vi "_NiFpga_HdlFifo_GetStream.vi"(7 "NUM_DMA_CHANNELS":u32=64, 11 "Fifo Number":u32) -> (3 "Fifo Stream":u32)   [LabVIEW 2023]
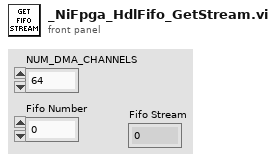
[diagram p1: front panel]
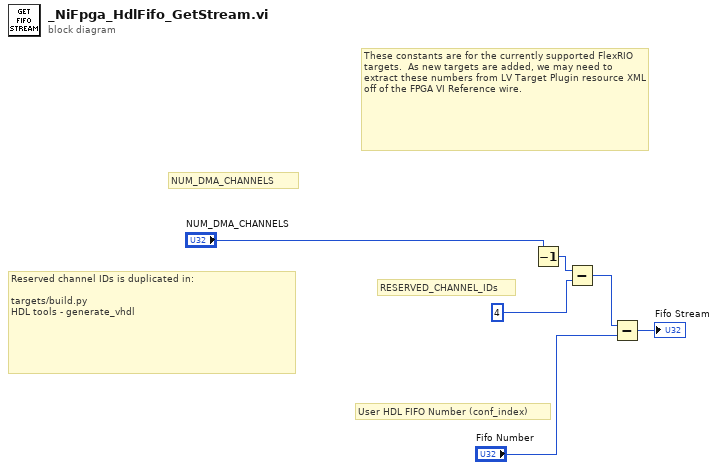
[diagram p0: block diagram]
diagram:
  # "Reserved channel IDs is duplicated in:\n\ntargets/build.py\nHDL tools - generate_vhdl"
  # "These constants are for the currently supported FlexRIO targets.  As new targets are added, we may need to extract these numbers from LV Target Plugin resource XML off of the FPGA VI Reference wire."
  # "NUM_DMA_CHANNELS"
  # "User HDL FIFO Number (conf_index)"
  # "RESERVED_CHANNEL_IDs"
  n1 = Decrement(x="NUM_DMA_CHANNELS") -> (x-1=w3:u32)
  n2 = Subtract(x=w3, y=u32 4 ("bytesPerElement")) -> (x-y=w6:u32)
  n3 = Subtract(x=w6, y="Fifo Number") -> (x-y=→"Fifo Stream":u32)
